vi "Check Username.vi"(8 "error in (no error)":errorcluster, 11 "[V] Login in":refnum<class "[V] Login.lvclass">) -> (0 "error out":errorcluster, 2 "username":string, 3 "[V] Login out":refnum<class "[V] Login.lvclass">)   [LabVIEW 2020, in "[V] Login.lvlib" / "[V] Login.lvclass"]
uses:
  [V] Login.lvclass
  [V] Login.lvclass/[V] Login.ctl
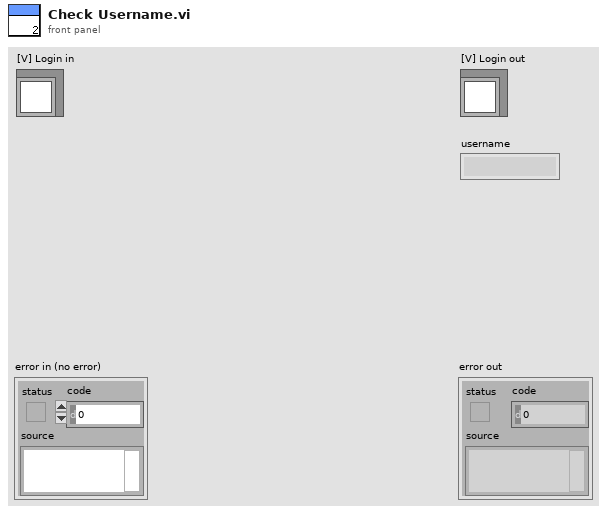
[diagram p1: front panel]
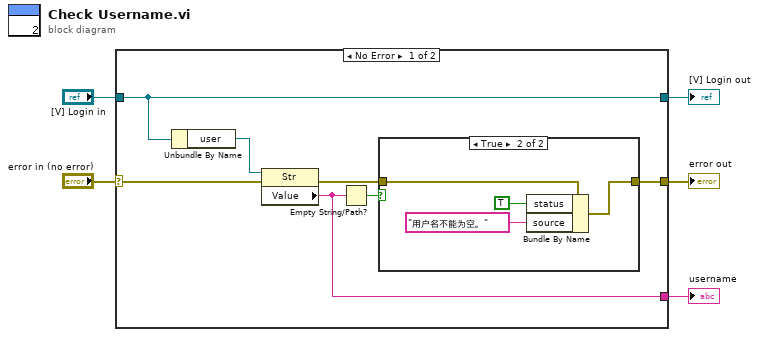
[diagram p0: block diagram]
diagram:
  n1 = case shown="No Error" "error in (no error)" {
    selector: "error in (no error)" -> [w11 w19]
    tunnel: [w6 w19] -> w4
    tunnel: [w12 w18] -> w2
    tunnel: "[V] Login in" -> [w12 w18]
    tunnel: [w9 _] -> w1
    frame No Error {
      n2 = Unbundle By Name(w12) -> ("user"=w10:refnum<vi>)
      n3 = property class="Str"(reference=w10, error in=w11) -> (error out=w7:errorcluster, "Value"=w9:string)  [unwired: 1 out]
      n4 = Empty String/Path?(string/path=w9) -> (empty?=w8:bool)
      n5 = case shown="True" w8 {
        tunnel: w7 -> [w13 w17]
        tunnel: [w13 w14] -> w6
        frame False {
        }
        frame True {
          n6 = Bundle By Name(cluster=w17, "status"=TRUE, "source"="用户名不能为空。") -> (w14:errorcluster)
        }
      }
    }
    frame Error {
    }
  }
  "error out" <- w4
  "[V] Login out" <- w2
  "username" <- w1
